vi "RS232_Handle.vi"(0 "Config":T1={"VISA resource name"="COM1", "baud rate"=9600, "data bits"=8, "parity"=0, "stop bits"=10} {"stop bits" items=["1.0"=10, "1.5"=15, "2.0"=20]; "parity" items=["None", "Odd", "Even", "Mark", "Space"]; "data bits" min=5 max=8 step=1}, 2 "Handle":enum16{"Open", "Read", "Wite", "Close"}(ring)=enum."Read", 7 "data in":string, 11 "error in":errorcluster) -> (6 "data out":string, 15 "error out":errorcluster={"status"=TRUE, "code"=-1073807339, "source"="VISA Read in RS232_Handle.vi->RS232_Hook.vi->COM-RS232Test.vi"})   [LabVIEW 2011]
uses:
  <vilib>/Instr/_visa.llb/VISA Configure Serial Port (Instr).vi
panel:
  in  "XON Character":u8=17 format="%.0x"
  in  "XOFF Character":u8=19 format="%.0x"
  in  "flow control":u16(ring) items=["None"=0, "XON/XOFF"=1, "RTS/CTS"=2, "DTR/DSR"=4]
  in  "End write with termination character?":bool
  in  "Input\nbuffer size":u32=4096
  in  "termination char\n(0xA = '\\n' = LF)":u8=10 format="%.0x"
  in  "End read on termination character?":bool
  in  "timeout (ms)":u32=100
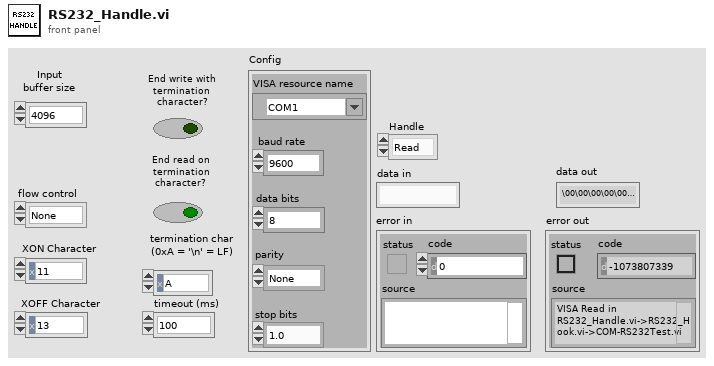
[diagram p1: front panel]
types:
  T1 = cluster{"VISA resource name":refnum<visa-resource-name>, "baud rate":u32, "data bits":u16, "parity":u16, "stop bits":u16}
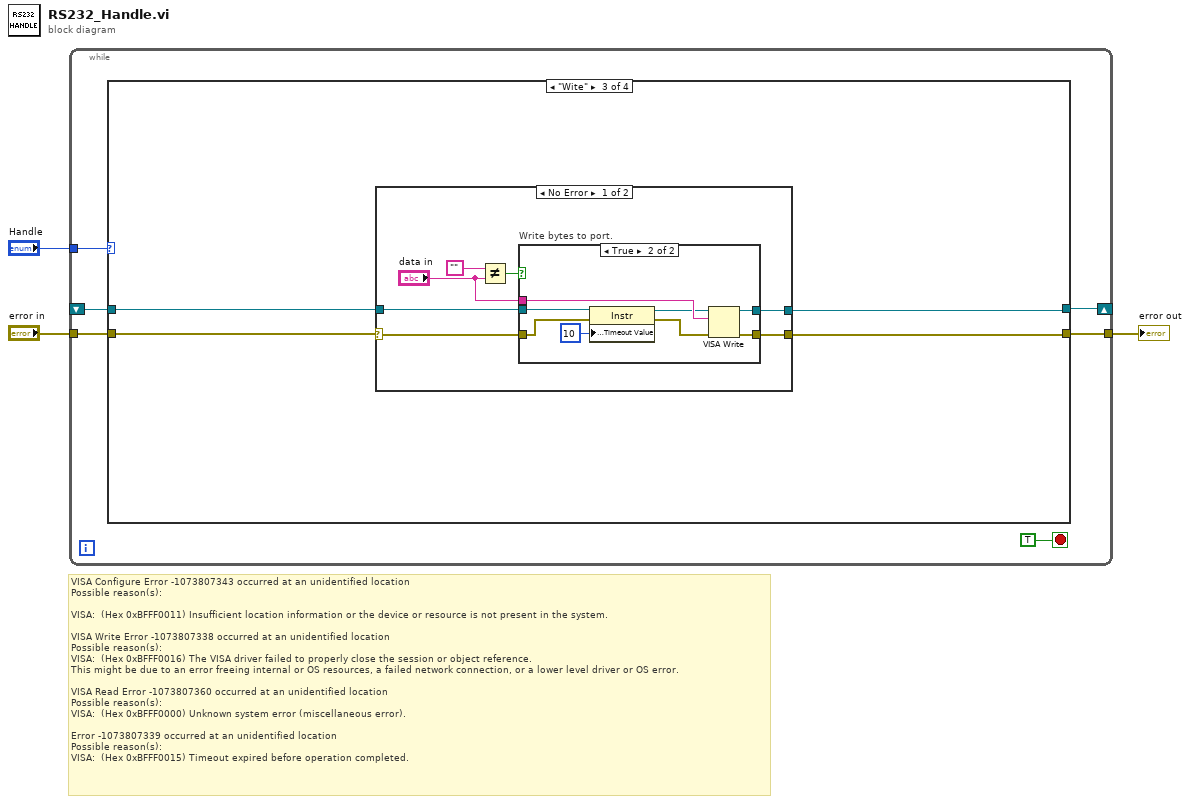
[diagram p0: block diagram]
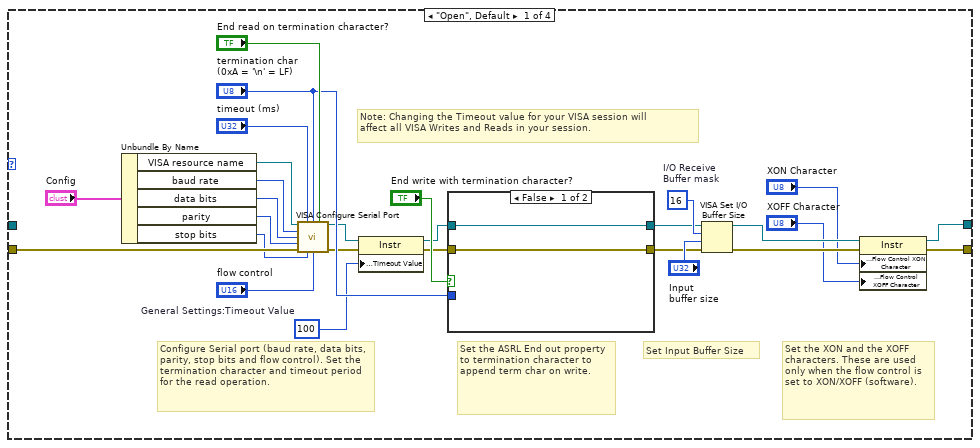
[diagram p2: hidden frame]
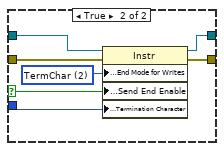
[diagram p3: hidden frame]
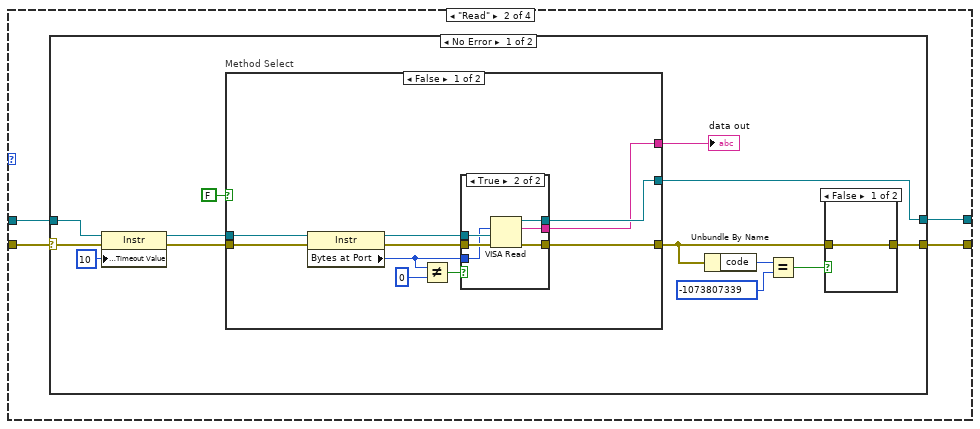
[diagram p4: hidden frame]
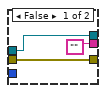
[diagram p5: hidden frame]
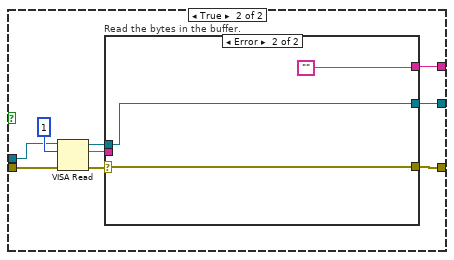
[diagram p6: hidden frame]
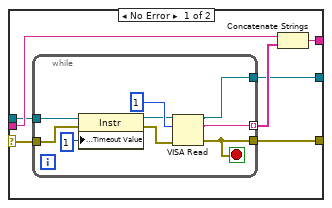
[diagram p7: hidden frame]
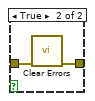
[diagram p8: hidden frame]
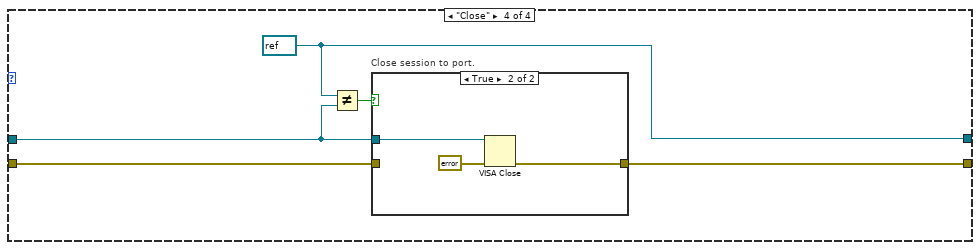
[diagram p12: hidden frame]
diagram:
  # "VISA Configure Error -1073807343 occurred at an unidentified location\nPossible reason(s):\n\nVISA:  (Hex 0xBFFF0011) Insufficient location information or the device or resource is not present in the system.\n\nVISA Write Error -1073807338 occurred at an unidentified location \nPossible reason(s):\nVISA:  (Hex 0xBFFF0016) The VISA driver failed to properly close the session or object reference. \nThis might be due to an error freeing internal or OS resources, a failed network connection, or a lower level driver or OS error.\n\nVISA Read Error -1073807360 occurred at an unidentified location\nPossible reason(s):\nVISA:  (Hex 0xBFFF0000) Unknown system error (miscellaneous error).\n\nError -1073807339 occurred at an unidentified location\nPossible reason(s):\nVISA:  (Hex 0xBFFF0015) Timeout expired before operation completed."
  n1 = while {
    tunnel: "Handle" -> [w9]
    tunnel: "error in" -> [w8]
    tunnel: [w6] -> w1
    shift-right: [w5] -> _
    shift-left: _ -> [w4]
    stop <- TRUE stop-if-true
    n2 = case shown="\"Wite\"" w9 {
      tunnel: w8 -> [w23 w47 w117 w142]
      tunnel: [w22 w46 w118 w141] -> w6
      tunnel: [w21 w48 w115 w138] -> w5
      tunnel: w4 -> [_ w49 w116 w140]
      frame "Open", Default {
        w14 = u32 100  # General Settings:Timeout Value
        w34 = u16 16  # I/O Receive Buffer mask
        # "Note: Changing the Timeout value for your VISA session will \naffect all VISA Writes and Reads in your session."
        # "Set the XON and the XOFF characters. These are used only when the flow control is set to XON/XOFF (software)."
        # "Configure Serial port (baud rate, data bits, parity, stop bits and flow control). Set the termination character and timeout period for the read operation."
        # "Set Input Buffer Size"
        # "Set the ASRL End out property to termination character to append term char on write."
        n3 = Unbundle By Name("Config") -> ("VISA resource name"=w19:refnum<visa-resource-name>, "baud rate"=w18:u32, "data bits"=w17:u16, "parity"=w16:u16, "stop bits"=w15:u16)
        n4 = call-poly "VISA Configure Serial Port"("VISA resource name"=w19, "timeout (10sec)"="timeout (ms)", "termination char\n(0xA = '\\n' = LF)"="termination char\n(0xA = '\\n' = LF)", "Enable Termination\nChar (T)"="End read on termination character?", "baud rate (9600)"=w18, "data bits (8)"=w17, "parity (0:none)"=w16, "error in (no error)"=w23, "stop bits (10: 1 bit)"=w15, "flow control (0:none)"="flow control") -> ("VISA resource name out"=w11:refnum<visa-resource-name>, "error out"=w13:errorcluster)  [unwired: 4 out]
        n5 = property class="Instr"(reference=w11, error in=w13, "General Settings:Timeout Value"=w14) -> (reference out=w10:refnum<visa-resource-name>, error out=w12:errorcluster)
        n6 = case shown="False" "End write with termination character?" {
          selector: "End write with termination character?" -> [_ w39]
          tunnel: w10 -> [w37 w45]
          tunnel: w12 -> [w38 w44]
          tunnel: [w37 w43] -> w24
          tunnel: [w38 w42] -> w25
          tunnel: "termination char\n(0xA = '\\n' = LF)" -> [_ w40]
          frame False {
          }
          frame True {
            w41 = u16 2 items=["None", "LastBit", "TermChar", "Break"] ("Serial Settings:Serial End Mode for Writes")
            n7 = property class="Instr"(reference=w45, error in=w44, "Serial Settings:End Mode for Writes"=w41, "Message Based Settings:Send End Enable"=w39, "Message Based Settings:Termination Character"=w40) -> (reference out=w43:refnum<visa-resource-name>, error out=w42:errorcluster)
          }
        }
        n8 = VISA Set I/O Buffer Size(VISA resource name=w24, mask (16)=w34, size (4096)="Input\nbuffer size", error in (no error)=w25) -> (VISA resource name out=w29:refnum<visa-resource-name>, error out=w28:errorcluster)
        n9 = property class="Instr"(reference=w29, error in=w28, "Serial Settings:Flow Control XON Character"="XON Character", "Serial Settings:Flow Control XOFF Character"="XOFF Character") -> (reference out=w21:refnum<visa-resource-name>, error out=w22:errorcluster)
      }
      frame "Read" {
        n10 = case shown="No Error" w47 {
          selector: w47 -> [w55 w113]
          tunnel: w49 -> [w56 w114]
          tunnel: [w52 w114] -> w48
          tunnel: [w61 w113] -> w46
          frame No Error {
            n11 = property class="Instr"(reference=w56, error in=w55, "General Settings:Timeout Value"=u32 10) -> (reference out=w58:refnum<visa-resource-name>, error out=w57:errorcluster)
            n12 = case "Method Select" shown="False" FALSE {
              tunnel: w58 -> [w72 w89]
              tunnel: w57 -> [w71 w88]
              tunnel: [w66 w84] -> w53
              tunnel: [w67 w83] -> w52
              tunnel: [w68 w82] -> w51
              frame False {
                n13 = property class="Instr"(reference=w72, error in=w71) -> (reference out=w70:refnum<visa-resource-name>, error out=w69:errorcluster, "Bytes at Port"=w63:u32)
                n14 = Not Equal?(x=w63, y=u32 0) -> (x != y?=w64:bool)
                n15 = case shown="True" w64 {
                  tunnel: w70 -> [w74 w81]
                  tunnel: w69 -> [w73 w80]
                  tunnel: [w73 w79] -> w68
                  tunnel: [w74 w78] -> w67
                  tunnel: ["" w77] -> w66
                  tunnel: w63 -> [_ w76]
                  frame False {
                  }
                  frame True {
                    n16 = VISA Read(VISA resource name=w81, byte count=w76, error in (no error)=w80) -> (VISA resource name out=w78:refnum<visa-resource-name>, read buffer=w77:string, error out=w79:errorcluster)  [unwired: 1 out]
                  }
                }
              }
              frame True {
                n17 = VISA Read(VISA resource name=w89, byte count=u32 1, error in (no error)=w88) -> (VISA resource name out=w85:refnum<visa-resource-name>, read buffer=w86:string, error out=w87:errorcluster)  [unwired: 1 out]
                n18 = case "Read the bytes in the buffer." shown="Error" w87 {
                  selector: w87 -> [w97 w108]
                  tunnel: w86 -> [w94 _]
                  tunnel: [w93 w107] -> w83
                  tunnel: [w96 ""] -> w84
                  tunnel: [w92 w108] -> w82
                  tunnel: w85 -> [w91 w107]
                  frame No Error {
                    n19 = while {
                      tunnel: w97 -> [w98]
                      tunnel: [w105] -> w93
                      tunnel: [w103] -> w95 mode=indexing
                      tunnel: [w106] -> w92
                      tunnel: w91 -> [w102]
                      stop <- w106 stop-if-true
                      n20 = property class="Instr"(reference=w102, error in=w98, "General Settings:Timeout Value"=u32 1) -> (reference out=w101:refnum<visa-resource-name>, error out=w100:errorcluster)
                      n21 = VISA Read(VISA resource name=w101, byte count=u32 1, error in (no error)=w100) -> (VISA resource name out=w105:refnum<visa-resource-name>, read buffer=w103:string, error out=w106:errorcluster)  [unwired: 1 out]
                    }
                    n22 = Concatenate Strings(w94, w95) -> (w96:string)
                  }
                  frame Error {
                  }
                }
              }
            }
            "data out" <- w53
            n23 = Unbundle By Name(w51) -> ("code"=w62:i32)
            n24 = Equal?(x=w62, y=-1073807339) -> (x = y?=w59:bool)
            n25 = case shown="False" w59 {
              tunnel: [w110 w112] -> w61
              tunnel: w51 -> [w110 w111]
              frame False {
              }
              frame True {
                n26 = call <vilib>:"Clear Errors.vi"("error in (no error)"=w111) -> ("error out"=w112:errorcluster)  [unwired: 6 in]
              }
            }
          }
          frame Error {
          }
        }
      }
      frame "Wite" {
        n27 = case shown="No Error" w117 {
          selector: w117 -> [w124 w137]
          tunnel: [w125 w137] -> w118
          tunnel: w116 -> [w123 w136]
          tunnel: [w122 w136] -> w115
          frame No Error {
            n28 = Not Equal?(x="", y="data in") -> (x != y?=w120:bool)
            n29 = case "Write bytes to port." shown="True" w120 {
              tunnel: [w126 w135] -> w125
              tunnel: w124 -> [w126 w130]
              tunnel: w123 -> [w127 w132]
              tunnel: [w127 w134] -> w122
              tunnel: "data in" -> [_ w133]
              frame False {
              }
              frame True {
                n30 = property class="Instr"(reference=w132, error in=w130, "General Settings:Timeout Value"=u32 10) -> (reference out=w131:refnum<visa-resource-name>, error out=w128:errorcluster)
                n31 = VISA Write(VISA resource name=w131, write buffer=w133, error in (no error)=w128) -> (VISA resource name out=w134:refnum<visa-resource-name>, error out=w135:errorcluster)  [unwired: 1 out]
              }
            }
          }
          frame Error {
          }
        }
      }
      frame "Close" {
        w138 = refnum<visa-resource-name> refnum ("VISA resource name out")
        n32 = Not Equal?(x=w138, y=w140) -> (x != y?=w139:bool)
        n33 = case "Close session to port." shown="True" w139 {
          tunnel: w142 -> [w143 _]
          tunnel: [w143 w146] -> w141
          tunnel: w140 -> [_ w145]
          frame False {
          }
          frame True {
            n34 = VISA Close(VISA resource name=w145, error in (no error)=errorcluster {"status"=FALSE, "code"=0, "source"=""} ("error constant")) -> (error out=w146:errorcluster)
          }
        }
      }
    }
  }
  "error out" <- w1
